vi "Read CEID File.vi"(8 "error in":errorcluster) -> (0 "error out":errorcluster, 3 "CEID Data":T1[](array[typedef]))   [LabVIEW 2020, in "SECS Communication.lvlib" / "SECS Data Class.lvclass"]
uses:
  SECS Data Class.lvclass
  CEID Data.ctl
  <vilib>/DATA AHEAD/XLR8/functions/Workbook/Open Create Workbook XLSX.vi
  <vilib>/DATA AHEAD/XLR8/XLR8.lvlib
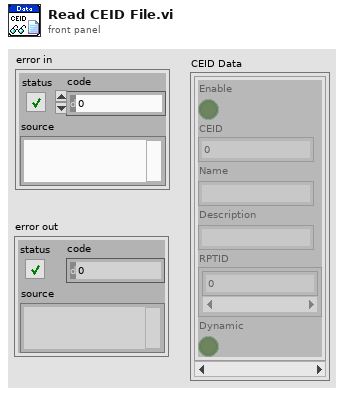
[diagram p1: front panel]
types:
  T1 = typedef "SECS Communication.lvlib/SECS Data Class.lvclass/CEID Data.ctl" = cluster{"Enable":bool, "CEID":u32, "Name":string, "Description":string, "RPTID":u32[], "Dynamic":bool}
  T2 = typedef "XLR8.lvlib/XLR8_Ref.ctl" = cluster{"WBK":refnum<k24>, "CurSheet":refnum<k24>, "File":refnum<k24>, "file path":string, "sheet":string, "Sheets":refnum<k24>[], "IsXML":bool, "Policy":i32}
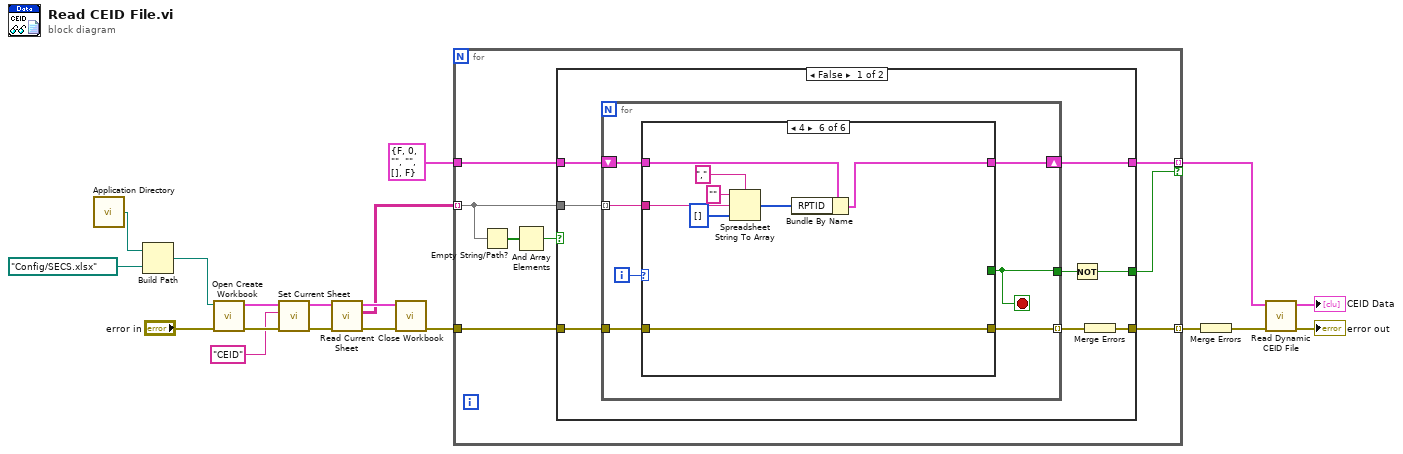
[diagram p0: block diagram]
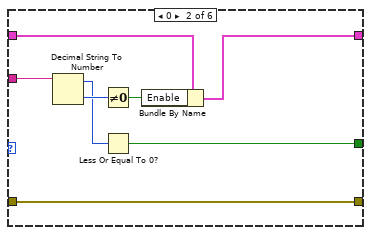
[diagram p3: hidden frame]
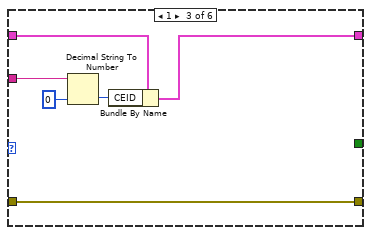
[diagram p4: hidden frame]
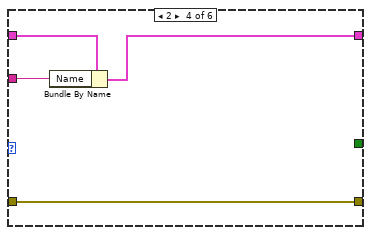
[diagram p5: hidden frame]
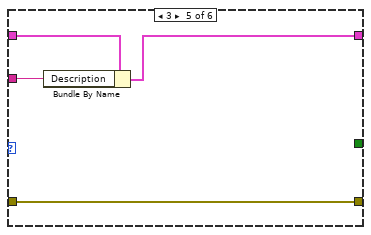
[diagram p6: hidden frame]
diagram:
  n1 = call <vilib>:"Application Directory.vi"() -> ("Application Directory"=w19:path)
  n2 = Build Path(base path=w19, name or relative path=path "Config/SECS.xlsx") -> (appended path=w1:path)
  n3 = call-poly <vilib>:"Open Create Workbook.vi"("error in"="error in", "Workbook Path"=w1) -> ("error out"=w15:errorcluster, "Refs Out"=w16:T2)  [unwired: 8 in]
  n4 = call <vilib>:"Set Current Sheet.vi"("error in"=w15, "Sheet to switch to"="CEID", "Refs In"=w16) -> ("error out"=w12:errorcluster, "Refs Out"=w13:T2)  [unwired: 7 in]
  n5 = call <vilib>:"Read Current Sheet.vi"("error in"=w12, "Refs In"=w13) -> ("error out"=w10:errorcluster, "Sheet-data out"=w8:string[][], "Refs Out"=w11:T2)  [unwired: 7 in]
  n6 = call <vilib>:"Close Workbook.vi"("error in"=w10, "Refs In"=w11) -> ("error out"=w9:errorcluster)  [unwired: 8 in, 1 out]
  n7 = for {
    tunnel: w9 -> [w24]
    tunnel: w8 -> [w25] mode=indexing
    tunnel: T1 {"Enable"=FALSE, "CEID"=0, "Name"="", "Description"="", "RPTID"=[], "Dynamic"=FALSE} ("CEID Data") -> [w23]
    tunnel: [w22] -> w4 mode=indexing if=w20
    tunnel: [w21] -> w7 mode=indexing
    n8 = Empty String/Path?(string/path=w25) -> (empty?=w27:bool[])
    n9 = And Array Elements(Boolean array=w27) -> (logical AND=w26:bool)
    n10 = case shown="False" w26 {
      tunnel: w25 -> [w35 _]
      tunnel: w24 -> [w32 w75]
      tunnel: w23 -> [w34 w76]
      tunnel: [w33 w76] -> w22
      tunnel: [w30 w75] -> w21
      tunnel: [w28 _] -> w20
      frame False {
        n11 = for {
          tunnel: w35 -> [w40] mode=indexing
          shift-right: [w39] -> w33
          shift-left: w34 -> [w42]
          tunnel: w32 -> [w38]
          tunnel: [w37] -> w31 mode=indexing
          tunnel: [w36] -> w29
          i -> [w41]
          stop <- w36 stop-if-true
          n12 = case shown="4" w41 {
            tunnel: w42 -> [w44 w49 w58 w62 w66 w73]
            tunnel: w40 -> [_ w52 w57 w61 w65 w71]
            tunnel: [w44 w47 w54 w60 w64 w74] -> w39
            tunnel: w38 -> [w43 w50 w53 w59 w63 w72]
            tunnel: [w43 w50 w53 w59 w63 w72] -> w37
            tunnel: [_ w45 _ _ _ _] -> w36
            frame Default {
            }
            frame 0 {
              n13 = Decimal String To Number(string=w52) -> (offset past number=w46:i32, number=w51:i32)  [unwired: 2 in]
              n14 = Not Equal To 0?(x=w51) -> (x != 0?=w48:bool)
              n15 = Less Or Equal To 0?(x=w46) -> (x <= 0?=w45:bool)
              n16 = Bundle By Name(cluster=w49, "Enable"=w48) -> (w47:T1)
            }
            frame 1 {
              n17 = Decimal String To Number(string=w57, default (0L)=u32 0 ("default (0 I32)")) -> (number=w56:u32)  [unwired: 1 in, 1 out]
              n18 = Bundle By Name(cluster=w58, "CEID"=w56) -> (w54:T1)
            }
            frame 2 {
              n19 = Bundle By Name(cluster=w62, "Name"=w61) -> (w60:T1)
            }
            frame 3 {
              n20 = Bundle By Name(cluster=w66, "Description"=w65) -> (w64:T1)
            }
            frame 4 {
              n21 = Spreadsheet String To Array(delimiter (Tab)=",", format string="", spreadsheet string=w71, array type (2D Dbl)=u32[] [] ("RPTID")) -> (array=w67:u32[])
              n22 = Bundle By Name(cluster=w73, "RPTID"=w67) -> (w74:T1)
            }
          }
        }
        n23 = Not(x=w29) -> (.not. x?=w28:bool)
        n24 = Merge Errors(w31) -> (w30:errorcluster)
      }
      frame True {
      }
    }
  }
  n25 = Merge Errors(w7) -> (w5:errorcluster)
  n26 = call "Read Dynamic CEID File.vi"("error in (no error)"=w5, "CEID Data In"=w4) -> ("error out"=→"error out":errorcluster, "CEID Data Out"=→"CEID Data":T1[])  [unwired: 8 in]
